vi "pass.vi"(8 "Reset":bool, 9 "Pass Button":bool, 10 "Arm Up Sensor":bool, 11 "Ball Presence Sensor":bool) -> (0 "Finished?":bool=TRUE, 2 "Arm State":T1, 3 "Roller Speed":dbl)   [LabVIEW 2013]
uses:
  <vilib>/Rock Robotics/WPI/Solenoid/WPI_SolenoidValue.ctl
  Pass States.ctl
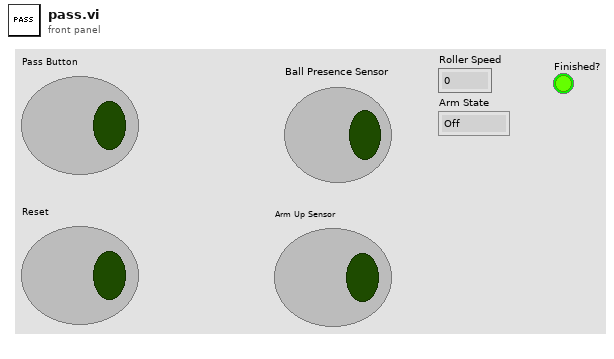
[diagram p1: front panel]
types:
  T1 = typedef "WPI_SolenoidValue.ctl" = enum16{"Off", "On", "Forward", "Reverse"}
  T2 = typedef "Pass States.ctl" = enum16{"Arm Down", "Release Ball", "Arm Up", "Finished"}
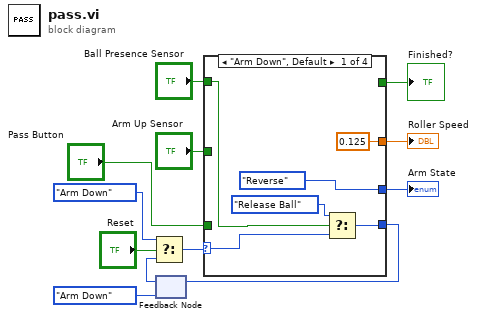
[diagram p0: block diagram]
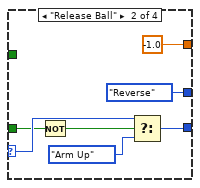
[diagram p2: hidden frame]
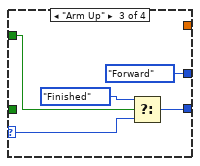
[diagram p3: hidden frame]
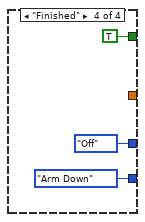
[diagram p4: hidden frame]
diagram:
  n1 = feedback #1(Pass_States."Arm Down" ("Enum")) -> (w5:T2)
  n2 = Select(t=Pass_States."Arm Down" ("Enum"), s="Reset", f=w5) -> (s? t:f=w4:T2)
  n3 = case shown="\"Arm Down\", Default" w4 {
    selector: w4 -> [w16 w21 w30 _]
    tunnel: "Ball Presence Sensor" -> [w13 _ _ _]
    tunnel: [0.125 -1.0 _ _] -> w11
    tunnel: [w18 w24 w27 Pass_States."Arm Down" ("Enum")] -> w6
    tunnel: "Arm Up Sensor" -> [_ _ w29 _]
    tunnel: [WPI_SolenoidValue."Reverse" ("Value") WPI_SolenoidValue."Reverse" ("Value") WPI_SolenoidValue."Forward" ("Value") WPI_SolenoidValue."Off" ("Value")] -> w8
    tunnel: [_ _ _ TRUE] -> w7
    tunnel: "Pass Button" -> [_ w20 _ _]
    frame "Arm Down", Default {
      n4 = Select(t=Pass_States."Release Ball" ("Enum"), s=w13, f=w16) -> (s? t:f=w18:T2)
    }
    frame "Release Ball" {
      n5 = Not(x=w20) -> (.not. x?=w19:bool)
      n6 = Select(t=w21, s=w19, f=Pass_States."Arm Up" ("Enum")) -> (s? t:f=w24:T2)
    }
    frame "Arm Up" {
      n7 = Select(t=Pass_States."Finished", s=w29, f=w30) -> (s? t:f=w27:T2)
    }
    frame "Finished" {
    }
  }
  "Roller Speed" <- w11
  "Arm State" <- w8
  "Finished?" <- w7
  n8 = feedback-in #1(w6) -> ()
